vi "Pressure Test.vi"() -> ()   [LabVIEW 2016]
uses:
  Q:/Common/LabVIEW GEA2 Toolkit/LabVIEW_GEA2_Toolkit.lvlibp/type defs/Source_Destination.ctl
  Q:/Common/LabVIEW GEA2 Toolkit/LabVIEW_GEA2_Toolkit.lvlibp/type defs/ERD Read Data In.ctl
  Q:/Common/LabVIEW GEA2 Toolkit/LabVIEW_GEA2_Toolkit.lvlibp/type defs/Data Type.ctl
  Q:/Common/LabVIEW GEA2 Toolkit/LabVIEW_GEA2_Toolkit.lvlibp
  Q:/Automation/Product Specific/Clothes Care/TL27/Projects/TL27.lvlib
panel:
  in  "Stop Button":bool
  out "Test Report":string
  out "Test Result":string
  out "Pressure Inches":string
  out "Hot Valve Status":string
  out "Cold Valve Status":string
  out "5+\"":bool
  out "4\"":bool
  out "3\"":bool
  out "2\"":bool
  out "1\"":bool
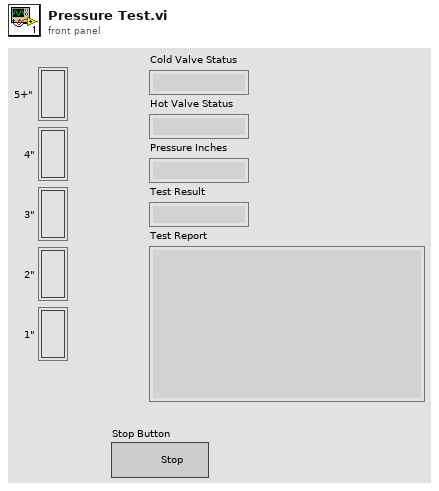
[diagram p1: front panel]
types:
  T1 = enum16{"ALL OFF", "Cold Valve", "Hot Valve", "Fabric Softener Valve", "Spray Rinse Valve", "Hot and Cold Valve"}
  T2 = typedef "LabVIEW_GEA2_Toolkit.lvlibp/ERD Read Data In.ctl" = cluster{"ERD Number":u16, "Data Type":T3}
  T3 = typedef "LabVIEW_GEA2_Toolkit.lvlibp/Data Type.ctl" = enum16{"string", "boolean", "uint8_t", "uint16_t", "uint32_t", "uint64_t", "int8_t", "int16_t", "int32_t", "int64_t"}
  T4 = typedef "LabVIEW_GEA2_Toolkit.lvlibp/Source_Destination.ctl" = cluster{"Source":u8, "Destination":u8}
  T5 = typedef "LabVIEW_GEA2_Toolkit.lvlibp/ERD Read Data Out.ctl" = cluster{"ERD Number":u16, "Data":string}
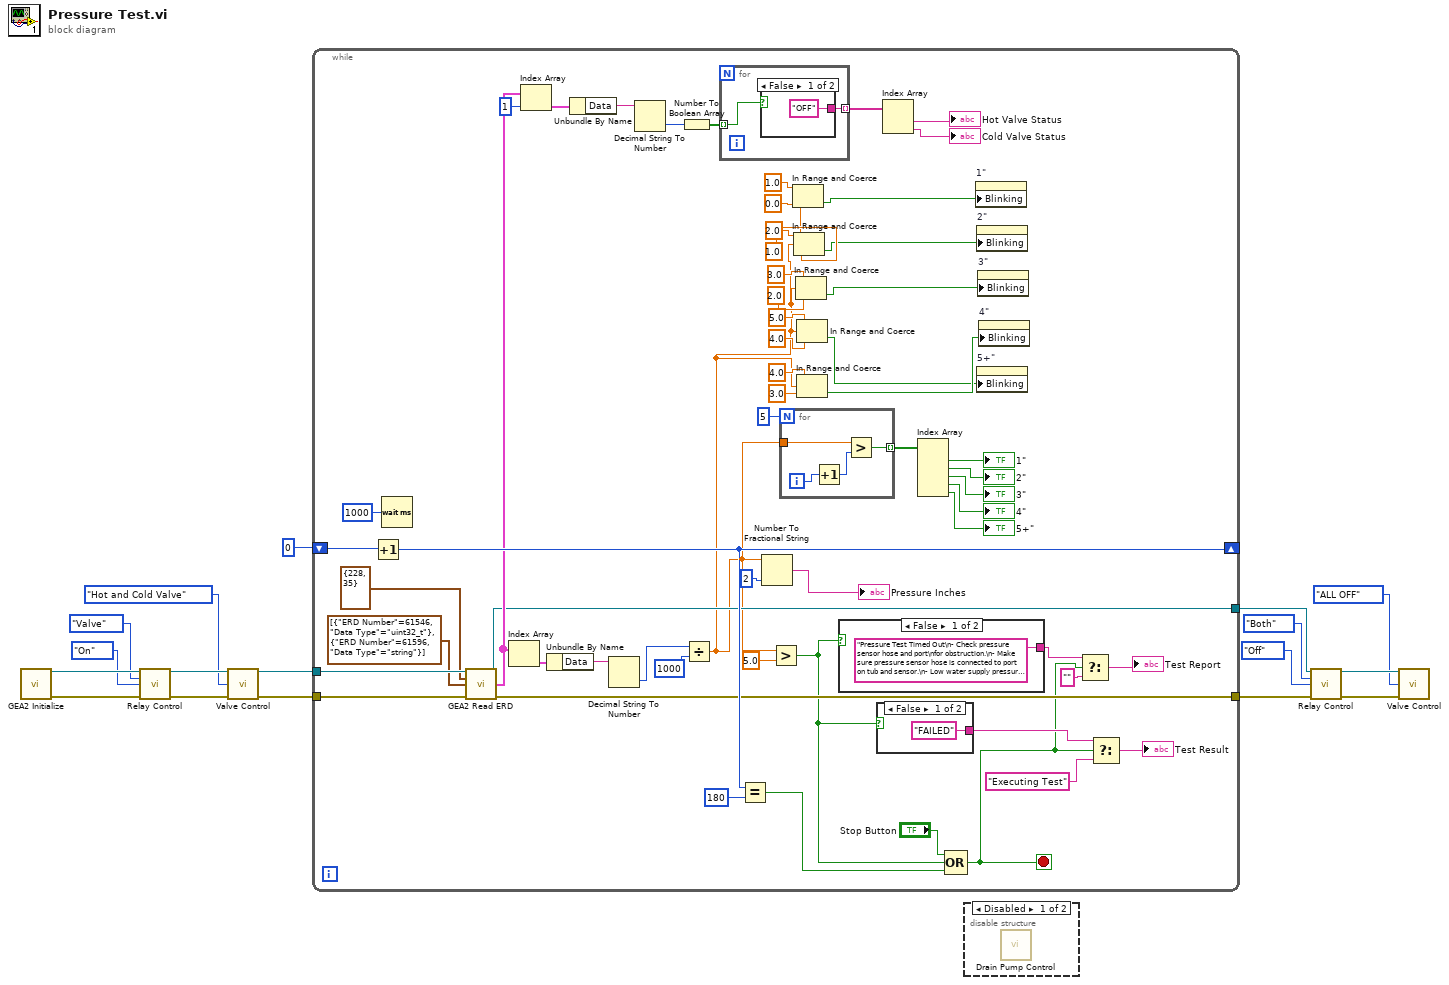
[diagram p0: block diagram]
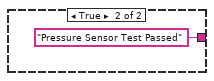
[diagram p3: hidden frame]
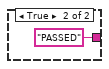
[diagram p4: hidden frame]
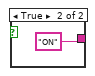
[diagram p5: hidden frame]
diagram:
  n1 = call "GEA2 Initialize.vi"() -> ("GEA2 Reference Out"=w15:refnum<k24>, "error out"=w17:errorcluster)  [unwired: 13 in, 1 out]
  n2 = call "Relay Control.vi"("GEA2 Reference In"=w15, "Relay"=enum16{"Motor Enable", "Valve", "Both"}."Valve", "State"=enum16{"On", "Off"}."On", "Error In"=w17) -> ("GEA2 Reference Out"=w14:refnum<k24>, "Error Out"=w16:errorcluster)  [unwired: 8 in, 2 out]
  n3 = call "Valve Control.vi"("GEA2 Reference In"=w14, "Fixed  Valve Control"=T1."Hot and Cold Valve", "Error In"=w16) -> ("GEA2 Reference Out"=w8:refnum<k24>, "Error Out"=w10:errorcluster)  [unwired: 11 in]
  n4 = while {
    tunnel: w10 -> [w71]
    shift-right: [w74] -> _
    shift-left: 0 -> [w75]
    tunnel: w8 -> [w70]
    tunnel: [w64] -> w2
    tunnel: [w23] -> w1
    stop <- w24 stop-if-true
    n5 = Increment(x=w75) -> (x+1=w74:i32)
    n6 = Wait (ms)(milliseconds to wait=u32 1000) -> ()  [unwired: 1 out]
    n7 = call "GEA2 Read ERD.vi"("GEA2 Reference In"=w70, "GEA Inputs"=T4 {"Source"=228, "Destination"=35}, "Read ERD List"=T2[] [{"ERD Number"=61546, "Data Type"=enum."uint32_t"}, {"ERD Number"=61596, "Data Type"=enum."string"}], "Error In"=w71) -> ("GEA2 Reference Out"=w23:refnum<k24>, "ERD Data Out"=w56:T5[], "Error Out"=w64:errorcluster)  [unwired: 8 in, 1 out]
    n8 = Index Array(array=w56) -> (element=w67:T5)  [unwired: 1 in]
    n9 = Index Array(array=w56, index=1) -> (element=w55:T5)
    n10 = Unbundle By Name(w67) -> ("Data"=w21:string)
    n11 = Unbundle By Name(w55) -> ("Data"=w54:string)
    n12 = Decimal String To Number(string=w21) -> (number=w53:i32)  [unwired: 2 in, 1 out]
    n13 = Decimal String To Number(string=w54) -> (number=w52:i32)  [unwired: 2 in, 1 out]
    n14 = Number To Boolean Array(number=w52) -> (Boolean array=w51:bool[])
    n15 = Divide(x=w53, y=1000) -> (x/y=w22:dbl)
    n16 = for {
      tunnel: w51 -> [w82] mode=indexing
      tunnel: [w81] -> w50 mode=indexing
      n17 = case shown="False" w82 {
        tunnel: ["OFF" "ON"] -> w81
        frame False {
        }
        frame True {
        }
      }
    }
    n18 = Equal?(x=w74, y=180) -> (x = y?=w72:bool)
    n19 = Number To Fractional String(number=w22, precision (6)=i16 2 ("width (-)")) -> (F-format string=→"Pressure Inches":string)  [unwired: 2 in]
    n20 = Greater?(x=w22, y=5.0) -> (0:w44:bool)
    n21 = for {
      N: 5 -> [_]
      tunnel: w22 -> [w86]
      tunnel: [w85] -> w62 mode=indexing
      i -> [w88]
      n22 = Increment(x=w88) -> (x+1=w87:i32)
      n23 = Greater?(x=w86, y=w87) -> (0:w85:bool)
    }
    n24 = In Range and Coerce(upper limit=1.0, x=w22, lower limit=0.0) -> (In Range?=w30:bool)  [unwired: 1 out]
    n25 = In Range and Coerce(upper limit=2.0, x=w22, lower limit=1.0) -> (In Range?=w29:bool)  [unwired: 1 out]
    n26 = In Range and Coerce(upper limit=3.0, x=w22, lower limit=2.0) -> (In Range?=w28:bool)  [unwired: 1 out]
    n27 = In Range and Coerce(upper limit=5.0, x=w22, lower limit=4.0) -> (In Range?=w26:bool)  [unwired: 1 out]
    n28 = In Range and Coerce(upper limit=4.0, x=w22, lower limit=3.0) -> (In Range?=w27:bool)  [unwired: 1 out]
    n29 = case shown="False" w44 {
      tunnel: ["Pressure Test Timed Out\n- Check pressure sensor hose and port\nfor obstruction.\n- Make sure pressure sensor hose is connected to port on tub and sensor.\n- Low water supply pressure can cause low fill volumes.  Check water supply.\n- Confirm operation of both the Hot and Cold valve using operate loads tab. " ("Test Result") "Pressure Sensor Test Passed" ("Test Result")] -> w43
      frame False {
      }
      frame True {
      }
    }
    n30 = case shown="False" w44 {
      tunnel: ["FAILED" ("Test Result") "PASSED" ("Test Result")] -> w47
      frame False {
      }
      frame True {
      }
    }
    n31 = Index Array(array=w50) -> (element #1=→"Hot Valve Status":string, element #2=→"Cold Valve Status":string)  [unwired: 2 in]
    n32 = Index Array(array=w62) -> (element #1=→"1\"":bool, element #2=→"2\"":bool, element #3=→"3\"":bool, element #4=→"4\"":bool, element #5=→"5+\"":bool)  [unwired: 5 in]
    n33 = Compound Arithmetic op=OR("Stop Button", w44, w72) -> (w24:bool)
    n34 = property on="1\"" class="Bool (strict)"("Blinking"=w30) -> ()  [unwired: 2 in, 2 out]
    n35 = property on="2\"" class="Bool (strict)"("Blinking"=w29) -> ()  [unwired: 2 in, 2 out]
    n36 = property on="5+\"" class="Bool (strict)"("Blinking"=w26) -> ()  [unwired: 2 in, 2 out]
    n37 = property on="3\"" class="Bool (strict)"("Blinking"=w28) -> ()  [unwired: 2 in, 2 out]
    n38 = property on="4\"" class="Bool (strict)"("Blinking"=w27) -> ()  [unwired: 2 in, 2 out]
    n39 = Select(t=w43, s=w24, f="") -> (s? t:f=→"Test Report":string)
    n40 = Select(t=w47, s=w24, f="Executing Test" ("Test Result")) -> (s? t:f=→"Test Result":string)
  }
  n41 = disable-structure shown="Disabled" {
    frame Disabled {
      n42 = call "Drain Pump Control.vi"() -> ()  [unwired: 14 in, 2 out]
    }
    frame Enabled {
    }
  }
  n43 = call "Relay Control.vi"("GEA2 Reference In"=w1, "Relay"=enum16{"Motor Enable", "Valve", "Both"}."Both", "State"=enum16{"On", "Off"}."Off", "Error In"=w2) -> ("GEA2 Reference Out"=w6:refnum<k24>, "Error Out"=w7:errorcluster)  [unwired: 8 in, 2 out]
  n44 = call "Valve Control.vi"("GEA2 Reference In"=w6, "Fixed  Valve Control"=T1."ALL OFF", "Error In"=w7) -> ()  [unwired: 11 in, 2 out]
